vi "Condition Private Data.vi"(8 "error in":errorcluster, 9 "PD Cluster":refnum<vi>, 10 "PD Control":refnum<vi>) -> (0 "error out":errorcluster)   [LabVIEW 2020, in "_Rescript.lvlib" / "Msg.lvlib" / "Msg.lvclass"]
uses:
  Msg.lvclass
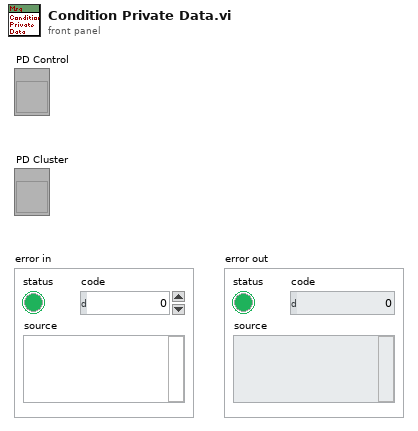
[diagram p1: front panel]
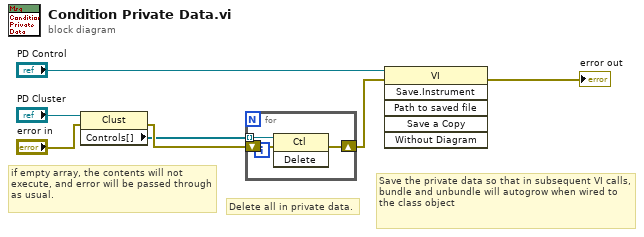
[diagram p0: block diagram]
diagram:
  # "if empty array, the contents will not execute, and error will be passed through as usual."
  # "Save the private data so that in subsequent VI calls, bundle and unbundle will autogrow when wired to the class object"
  # "Delete all in private data."
  n1 = property class="Clust"(reference="PD Cluster", error in="error in") -> (error out=w7:errorcluster, "Controls[]"=w4:refnum<vi>[])  [unwired: 1 out]
  n2 = for {
    tunnel: w4 -> [w10] mode=indexing
    shift-right: [w8] -> w1
    shift-left: w7 -> [w9]
    n3 = invoke class="Ctl" method="Delete"(reference=w10, error in=w9) -> (error out=w8:errorcluster)  [unwired: 1 in, 2 out]
  }
  n4 = invoke class="VI" method="Save.Instrument"(reference="PD Control", error in=w1) -> (error out=→"error out":errorcluster)  [unwired: 4 in, 5 out]
